vi "Read Config.vi"(8 "error in (no error)":errorcluster, 11 "Path":path) -> (0 "error out":errorcluster, 2 "Config":T1, 3 "File Created?":bool)   [LabVIEW 2023, in "VI Properties Editor.lvlib"]
uses:
  VI Properties Editor.lvlib
  CTLs/Config.ctl
  <vilib>/Utility/config.llb/Read Key (String).vi
  <vilib>/Utility/config.llb/Read Key (Boolean).vi
  <vilib>/Utility/config.llb/NI_LVConfig.lvlib
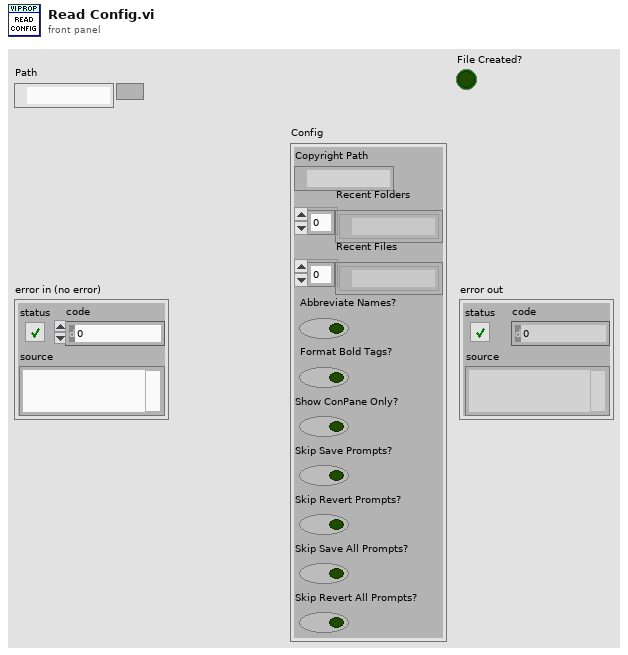
[diagram p1: front panel]
types:
  T1 = typedef "VI Properties Editor.lvlib/Config.ctl" = cluster{"Copyright Path":path, "Recent Folders":path[], "Recent Files":path[], "Abbreviate Names?":bool, "Format Bold Tags?":bool, "Show ConPane Only?":bool, "Skip Save Prompts?":bool, "Skip Revert Prompts?":bool, "Skip Save All Prompts?":bool, "Skip Revert All Prompts?":bool}
  T2 = typedef "NI_LVConfig.lvlib/Config Data RefNum.ctl" = refnum<k1>
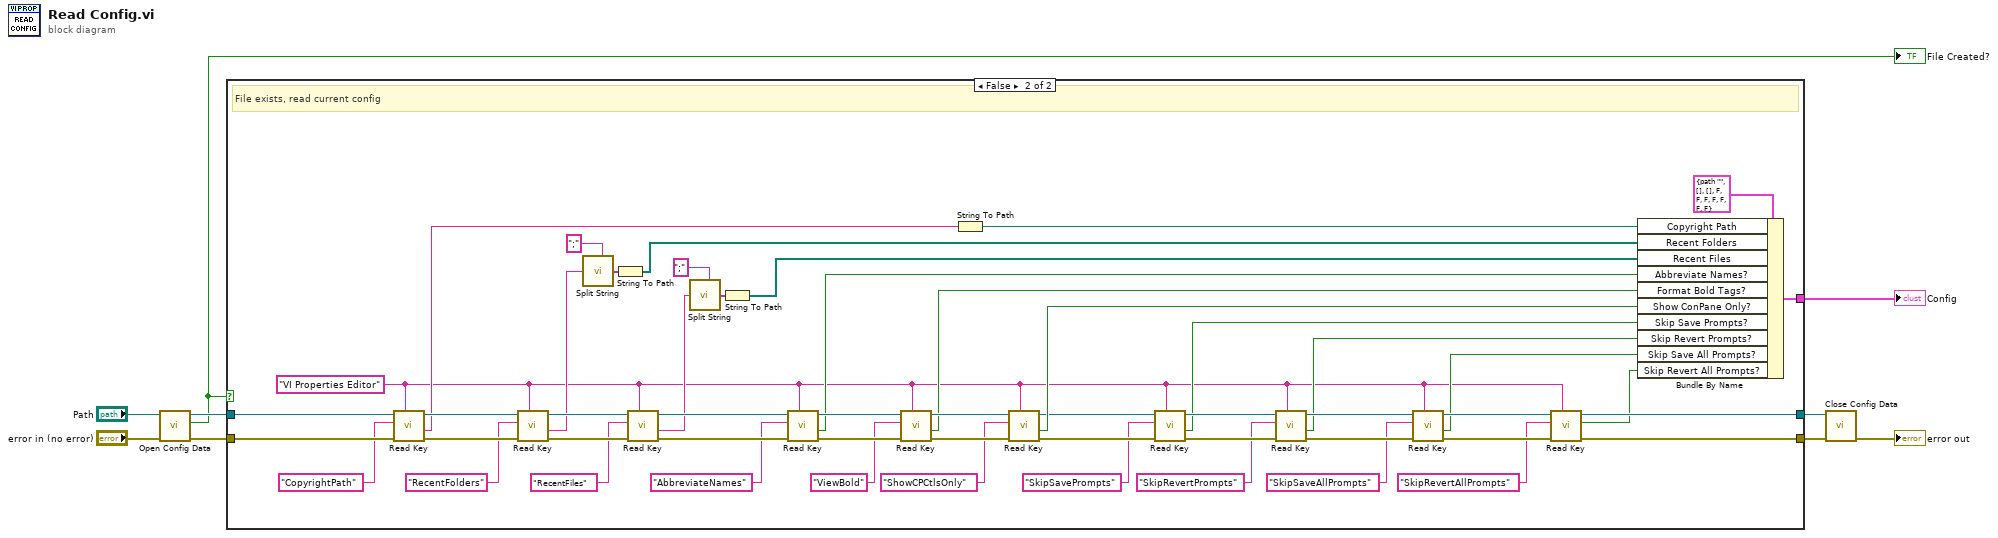
[diagram p0: block diagram]
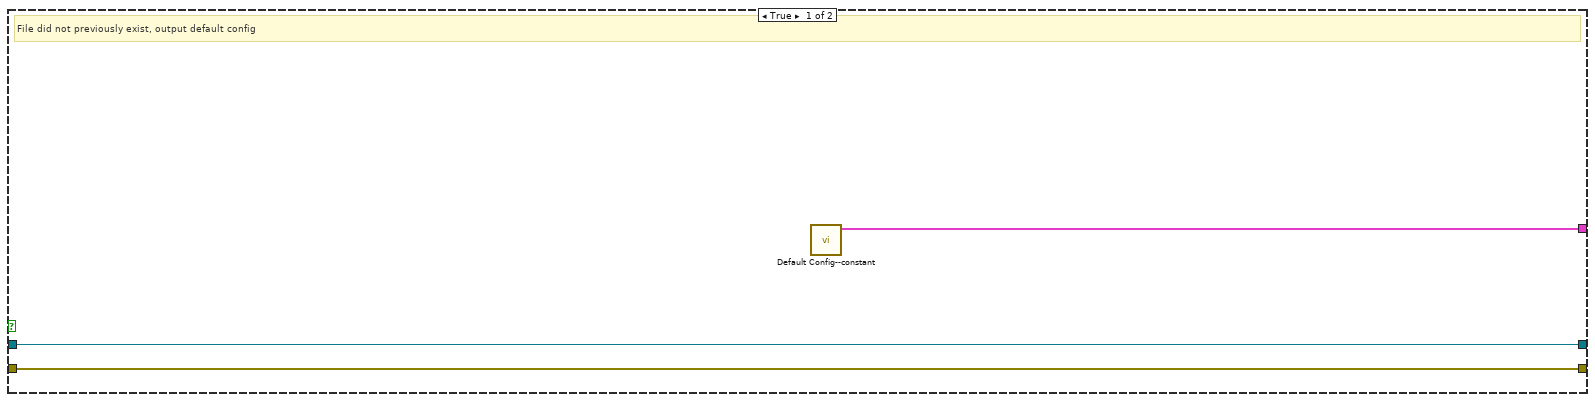
[diagram p2: hidden frame]
diagram:
  n1 = call <vilib>:"Open Config Data.vi"("error in (no error)"="error in (no error)", "configuration file path"="Path") -> ("error out"=w8:errorcluster, "file created?"=w2:bool, "refnum"=w4:T2)  [unwired: 7 in]
  "File Created?" <- w2
  n2 = case shown="False" w2 {
    tunnel: w4 -> [w10 w50]
    tunnel: w8 -> [w12 w64]
    tunnel: [w12 w16] -> w7
    tunnel: [w10 w15] -> w3
    tunnel: [w11 w43] -> w1
    frame True {
      # "File did not previously exist, output default config"
      n3 = call "Default Config--constant.vi"() -> ("Default Config"=w11:T1)  [unwired: 11 in]
    }
    frame False {
      w13 = "VI Properties Editor" ("section")
      # "File exists, read current config"
      n4 = call-poly <vilib>:"Read Key.vi"("section"=w13, "error in (no error)"=w64, "key"="CopyrightPath", "refnum"=w50) -> ("error out"=w61:errorcluster, "value"=w42:string, "refnum out"=w53:T2)  [unwired: 4 in, 1 out]
      n5 = call-poly <vilib>:"Read Key.vi"("section"=w13, "error in (no error)"=w61, "key"="RecentFolders", "refnum"=w53) -> ("error out"=w60:errorcluster, "value"=w36:string, "refnum out"=w52:T2)  [unwired: 4 in, 1 out]
      n6 = call <vilib>:"Split String.vi"("Split Pattern"=";", "Input String"=w36) -> ("Split String"=w35:string[])  [unwired: 5 in]
      n7 = String To Path(string=w35) -> (path=w34:path[])
      n8 = call-poly <vilib>:"Read Key.vi"("section"=w13, "error in (no error)"=w60, "key"="RecentFiles", "refnum"=w52) -> ("error out"=w59:errorcluster, "value"=w31:string, "refnum out"=w51:T2)  [unwired: 4 in, 1 out]
      n9 = call <vilib>:"Split String.vi"("Split Pattern"=";", "Input String"=w31) -> ("Split String"=w33:string[])  [unwired: 5 in]
      n10 = String To Path(string=w33) -> (path=w30:path[])
      n11 = call-poly <vilib>:"Read Key.vi"("section"=w13, "error in (no error)"=w59, "key"="AbbreviateNames", "refnum"=w51) -> ("error out"=w63:errorcluster, "value"=w41:bool, "refnum out"=w47:T2)  [unwired: 4 in, 1 out]
      n12 = call-poly <vilib>:"Read Key.vi"("section"=w13, "error in (no error)"=w63, "key"="ViewBold", "refnum"=w47) -> ("error out"=w62:errorcluster, "value"=w40:bool, "refnum out"=w54:T2)  [unwired: 4 in, 1 out]
      n13 = String To Path(string=w42) -> (path=w45:path)
      n14 = call-poly <vilib>:"Read Key.vi"("section"=w13, "error in (no error)"=w62, "key"="ShowCPCtlsOnly", "refnum"=w54) -> ("error out"=w56:errorcluster, "value"=w28:bool, "refnum out"=w23:T2)  [unwired: 4 in, 1 out]
      n15 = call-poly <vilib>:"Read Key.vi"("section"=w13, "error in (no error)"=w56, "key"="SkipSavePrompts", "refnum"=w23) -> ("error out"=w58:errorcluster, "value"=w19:bool, "refnum out"=w22:T2)  [unwired: 4 in, 1 out]
      n16 = call-poly <vilib>:"Read Key.vi"("section"=w13, "error in (no error)"=w58, "key"="SkipRevertPrompts", "refnum"=w22) -> ("error out"=w55:errorcluster, "value"=w18:bool, "refnum out"=w21:T2)  [unwired: 4 in, 1 out]
      n17 = call-poly <vilib>:"Read Key.vi"("section"=w13, "error in (no error)"=w55, "key"="SkipSaveAllPrompts", "refnum"=w21) -> ("error out"=w57:errorcluster, "value"=w17:bool, "refnum out"=w20:T2)  [unwired: 4 in, 1 out]
      n18 = call-poly <vilib>:"Read Key.vi"("section"=w13, "error in (no error)"=w57, "key"="SkipRevertAllPrompts", "refnum"=w20) -> ("error out"=w16:errorcluster, "found?"=w14:bool, "refnum out"=w15:T2)  [unwired: 4 in, 1 out]
      n19 = Bundle By Name(cluster=T1 {"Copyright Path"=path "", "Recent Folders"=[], "Recent Files"=[], "Abbreviate Names?"=FALSE, "Format Bold Tags?"=FALSE, "Show ConPane Only?"=FALSE, "Skip Save Prompts?"=FALSE, "Skip Revert Prompts?"=FALSE, "Skip Save All Prompts?"=FALSE, "Skip Revert All Prompts?"=FALSE} ("Config"), "Copyright Path"=w45, "Recent Folders"=w34, "Recent Files"=w30, "Abbreviate Names?"=w41, "Format Bold Tags?"=w40, "Show ConPane Only?"=w28, "Skip Save Prompts?"=w19, "Skip Revert Prompts?"=w18, "Skip Save All Prompts?"=w17, "Skip Revert All Prompts?"=w14) -> (w43:T1)
    }
  }
  "Config" <- w1
  n20 = call <vilib>:"Close Config Data.vi"("error in (no error)"=w7, "refnum"=w3) -> ("error out"=→"error out":errorcluster)  [unwired: 8 in, 1 out]
